vi "Transmit.vi"(8 "error in (no error)":errorcluster, 11 "Framework in":refnum<class "Framework.lvclass">) -> (0 "error out":errorcluster, 3 "Framework out":refnum<class "Framework.lvclass">)   [LabVIEW 2017, in "DSF Core.lvlib" / "Framework.lvclass"]
uses:
  Framework.lvclass
  Framework.lvclass/Framework.ctl
  Performance/Performance.lvclass/Performance.ctl
  Plugin/Plugin.lvclass/Plugin.ctl
  Transfer Group/Transfer Group.lvclass/Transfer Group.ctl
  Timing/Timing.lvclass/Timing.ctl
  Buffer/Buffers.lvclass/Buffers.ctl
  <vilib>/NI/Memory Manager/Classes/Pointer/Pointer.lvclass/Pointer.ctl
  Interfaces/Interface/Interface.lvclass/Interface.ctl
  Performance/Write Tx Duration.vi
  Transfer Group/Wait For Previous.vi
  Transfer Group/Increment Iteration.vi
  Transfer Group/Copy Inline to Async.vi
  Transfer Group/Get Iteration.vi
  Dispatcher/Dispatch Transfer Group.vi
  Transfer Group/Get ID.vi
  Plugin/Get ID.vi
  Transfer Group/Get Active.vi
  <vilib>/NI/Memory Manager/Classes/Pointer/Write.vi
  <vilib>/NI/Memory Manager/Classes/Pointer/Write U32.vi
  Transfer Group/Retrieve from FIFO.vi
  Timing/Increment Iteration.vi
  Buffer/Copy Inline to Async.vi
  Timing/Get Iteration.vi
  Interfaces/Dispatcher/Send Command.vi
  <vilib>/NI/Memory Manager/Classes/Pointer/Write (No Check).vi
  <vilib>/NI/Memory Manager/Classes/Pointer/Write (No Check) U32.vi
  <vilib>/NI/Memory Manager/Classes/Pointer/Check Move.vi
  Transfer Group/Read Return FIFO.vi
  <vilib>/NI/Memory Manager/Classes/Pointer/Copy All.vi
  Interfaces/Dispatcher/Write.vi
  Interfaces/Dispatcher/Write Dispatcher Command.vi
  <vilib>/NI/Memory Manager/Classes/Pointer/Get Address.vi
  <vilib>/NI/Memory Manager/Classes/Pointer/Check Null Pointer.vi
  <vilib>/NI/Memory Manager/Classes/Pointer/Check Count.vi
  <vilib>/NI/Memory Manager/Classes/Pointer/Check Bounds (Power of 2).vi
  <vilib>/NI/Memory Manager/Classes/Pointer/Get Size.vi
  <vilib>/NI/Memory Manager/Classes/Pointer/Copy.vi
  Interfaces/Interface/Write Command.vi
  <vilib>/NI/Memory Manager/Classes/Pointer/Errors.vi
  <vilib>/NI/Memory Manager/Classes/Pointer/Null Pointer.vi
  <vilib>/NI/Memory Manager/Classes/Pointer/Is Null.vi
  <vilib>/NI/Memory Manager/Classes/Pointer/Out of Bounds.vi
  <vilib>/NI/Memory Manager/Classes/Pointer/Check Bounds.vi
  <vilib>/NI/Memory Manager/Classes/Pointer/Copy (No Check).vi
  <vilib>/NI/Memory Manager/Classes/Pointer/Check Pointer Bounds.vi
  Interfaces/Interface/Write RT FIFO.vi
  <vilib>/NI/Memory Manager/Classes/Pointer/Create Error.vi
  <vilib>/NI/Memory Manager/VIs/Source.Write.String.vi
  <vilib>/NI/Memory Manager/Classes/Pointer/Write Pointer Size.vi
  <vilib>/NI/Memory Manager/VIs/Source.Write.Scalar.Base10.vi
  <vilib>/NI/Memory Manager/VIs/Source.Write.Scalar.Base10 (U64).vi
  <vilib>/NI/Memory Manager/Classes/Pointer/Check Buffer Bounds.vi
  <vilib>/NI/Memory Manager/VIs/New Error Cluster Constant.vi
  <vilib>/NI/Memory Manager/VIs/New Error Cluster Constant (512B).vi
  <vilib>/NI/Memory Manager/VIs/Error Cluster.Set Status.vi
  <vilib>/NI/Memory Manager/VIs/Error Cluster.Set Code.vi
  <vilib>/NI/Memory Manager/VIs/Error Cluster.Set VI Source.vi
  <vilib>/NI/Memory Manager/Constants/Constants.vi
  <vilib>/NI/Memory Manager/Constants/Library Name.vi
  <vilib>/NI/Memory Manager/Classes/Pointer/Pointer Error Info.vi
  <vilib>/NI/Memory Manager/Constants/Pointer Class Name.vi
  <vilib>/NI/Memory Manager/Classes/Pointer/Buffer Underflow.vi
  Buffer/Buffer.lvclass
  C:/Program Files (x86)/National Instruments/LabVIEW 2017/vi.lib/NI/Memory Manager/Classes/Pointer/Pointer.lvclass
  Interfaces/Dispatcher/Dispatcher Interface.lvclass
  C:/Users/Admin/Desktop/Data Sharing Framework/Source/Core/Classes/Interfaces/Interface/Interface.lvclass
  Transfer Group/Update Status.vi
  Transfer Group/Errors.vi
  Transfer Group/Return Timeout Error.vi
  Transfer Group/Increment Late Count.vi
  Transfer Group/Invalid Iteration Error.vi
  Interfaces/Interface/Errors.vi
  Interfaces/Dispatcher/Command Timeout.vi
  Interfaces/Dispatcher/Class Name.vi
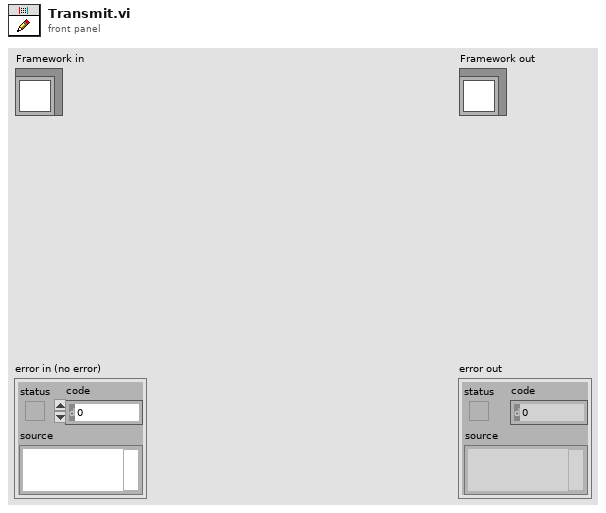
[diagram p1: front panel]
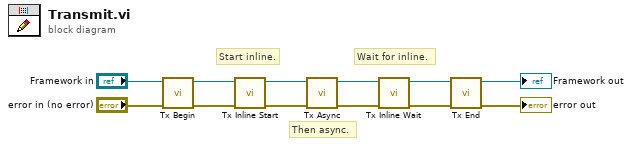
[diagram p0: block diagram]
diagram:
  # "Wait for inline."
  # "Start inline."
  # "Then async."
  n1 = call "Tx Begin.vi"("error in (no error)"="error in (no error)", "Framework in"="Framework in") -> ("error out"=w1:errorcluster, "Framework out"=w10:refnum<class "Framework.lvclass">)  [unwired: 8 in]
  n2 = call "Tx Inline Start.vi"("error in (no error)"=w1, "Framework in"=w10) -> ("error out"=w3:errorcluster, "Framework out"=w2:refnum<class "Framework.lvclass">)  [unwired: 8 in]
  n3 = call "Tx Async.vi"("error in (no error)"=w3, "Framework in"=w2) -> ("error out"=w5:errorcluster, "Framework out"=w4:refnum<class "Framework.lvclass">)  [unwired: 8 in]
  n4 = call "Tx Inline Wait.vi"("error in (no error)"=w5, "Framework in"=w4) -> ("error out"=w8:errorcluster, "Framework out"=w9:refnum<class "Framework.lvclass">)  [unwired: 8 in]
  n5 = call "Tx End.vi"("error in (no error)"=w8, "Framework in"=w9) -> ("error out"=→"error out":errorcluster, "Framework out"=→"Framework out":refnum<class "Framework.lvclass">)  [unwired: 8 in]
